vi "GEA_Brute_Force_SM.vi"(0 "ComPort":refnum<visa-resource-name>="COM1", 1 "Destination Address":u8=96 format="%.0x", 2 "Source Address":u8=128 format="%.0x", 5 "Command":u8(ring)=15 items=["CMD_WRITE_SETPOINTS", "RQST_NON_CRIT_VERSION", "RQST_CRIT_VERSION", "RQST_EEPROM_VERSION", "RQST_T2_RESISTANCE", "RQST_T3A_RESISTANCE", "RQST_T3B_RESISTANCE", "RQST_T4_RESISTANCE", "RQST_T5_RESISTANCE", "RQST_IDLB_RESISTANCE", "RQST_MODE_SELECT_RESISTANCE", "RQST_STATUS INFO", "RQST_SS_FAULT_COUNTS", "RQST_OTHER_FAULT_COUNTS", "CMD_CLEAR_FAULT_COUNTS", "RQST_HYPERTERM_OUTPUT_DATA", "RQST_READ_PERSONALITY", "RQST_DSM_OVERRIDE_STATUS", "RQST_STATUS_QUERY", "RQST_HEM_KWH_DATA", "RQST_SERVICE_ERROR_CODES", "RQST_OVERRIDE_STATUS", "CMD_CLEAR_OVERRIDE_STATUS", "CMD_CLEAR_ENERGY_USAGE_CTRS", "CMD_COMP_OFF", "CMD_UE_2_SECONDS", "CMD_LE_2_SECONDS", "CMD_COMP_ON", "CMD_HP_RUN_6MIN", "RQST_TEMP_RANGE", "RQST_VACATION_RANGE", "RQST_STD_ELEC_RANGE", "RQST_WATER_CAPACITY", "CMD_CANCEL_EEV_POSITION", "RQST_SUPPORTED_MODES", "CMD_CONTROL_FAN1", "CMD_EEV_POSITION", "CMD_SET_EEV_START_POSITION", "CMD_SET_EEV_STOP_POSITION", "CMD_UPDATE_DSM_LEVEL", "CMD_SET_PID_I_DENOMINATOR", "CMD_SET_PID_I_NUMERATOR", "RQST_DATA_FROM_MEMORY", "CMD_OVERRIDE_STATUS_CHANGED", "CMD_SET_PID_P_DENOMINATOR", "CMD_SET_PID_P_NUMERATOR", "CMD_SET_PID_RUN_SH_TARGET", "CMD_SET_PID_START_DWELL_TIME", "CMD_SET_PID_TRANSITION_TIME", "CMD_SET_PID_TRANS_SH_TARGET", "CMD_SET_PID_UPDATE_RATE", "RQST_DATA_FROM_DATA_FLASH", "CMD_DSM_OVERRIDES", "CMD_UPDATE_MODE", "CMD_UPDATE_SPECIAL_OPERATION", "CMD_SET_CURRENTS", "CMD_RESET_FILTER_TIMES", "CMD_TURN_ON_DLB", "RQST_PID_PARAMETERS", "CMD_CHECK_CRC", "CMD_ENTER_FACT_MODE", "CMD_RESET", "CMD_RESTORE_EEPROM_DEFAULTS"], 7 "Command Data":u8[](array[numeric]) format="%02x", 9 "InitSerial?":bool=TRUE, 11 "Error In":errorcluster) -> (4 "WriteACK":bool, 6 "Read_ACK":bool, 8 "DataReturned":u8[](array[numeric]) format="%.0x", 14 "CRC Match":bool, 15 "Error Out":errorcluster)   [LabVIEW 2009]
uses:
  <vilib>/Instr/_visa.llb/VISA Configure Serial Port (Instr).vi
  HEWH Error Enumeration.ctl
panel:
  out "tStart":i32
  out "Diff Time":i32[](array[numeric])
  out "Serial Settings:Number of Bytes at Serial Port":u32
  out "Time Array":i32[](array[numeric])
  out "ACK(E1?)":u8[](array[numeric]) format="%.0x"
  out "Local?":bool
  out "State Array":string[](array[string])
  out "CRCRead":u8[](array[numeric]) format="%.0x"
  out "Command":u8[](array[numeric])=[226, 96, 8, 128, 86, 123, 137, 227] format="%.0x"
  in  "Send HEWH Cmd":bool
  in  "Write Rand":bool
  in  "Random Data":u8[](array[numeric]) format="%.0x"
  out "WriteOK":bool
  out "ReadArray":u8[](array[numeric]) format="%.0x"
  in  "OK":bool
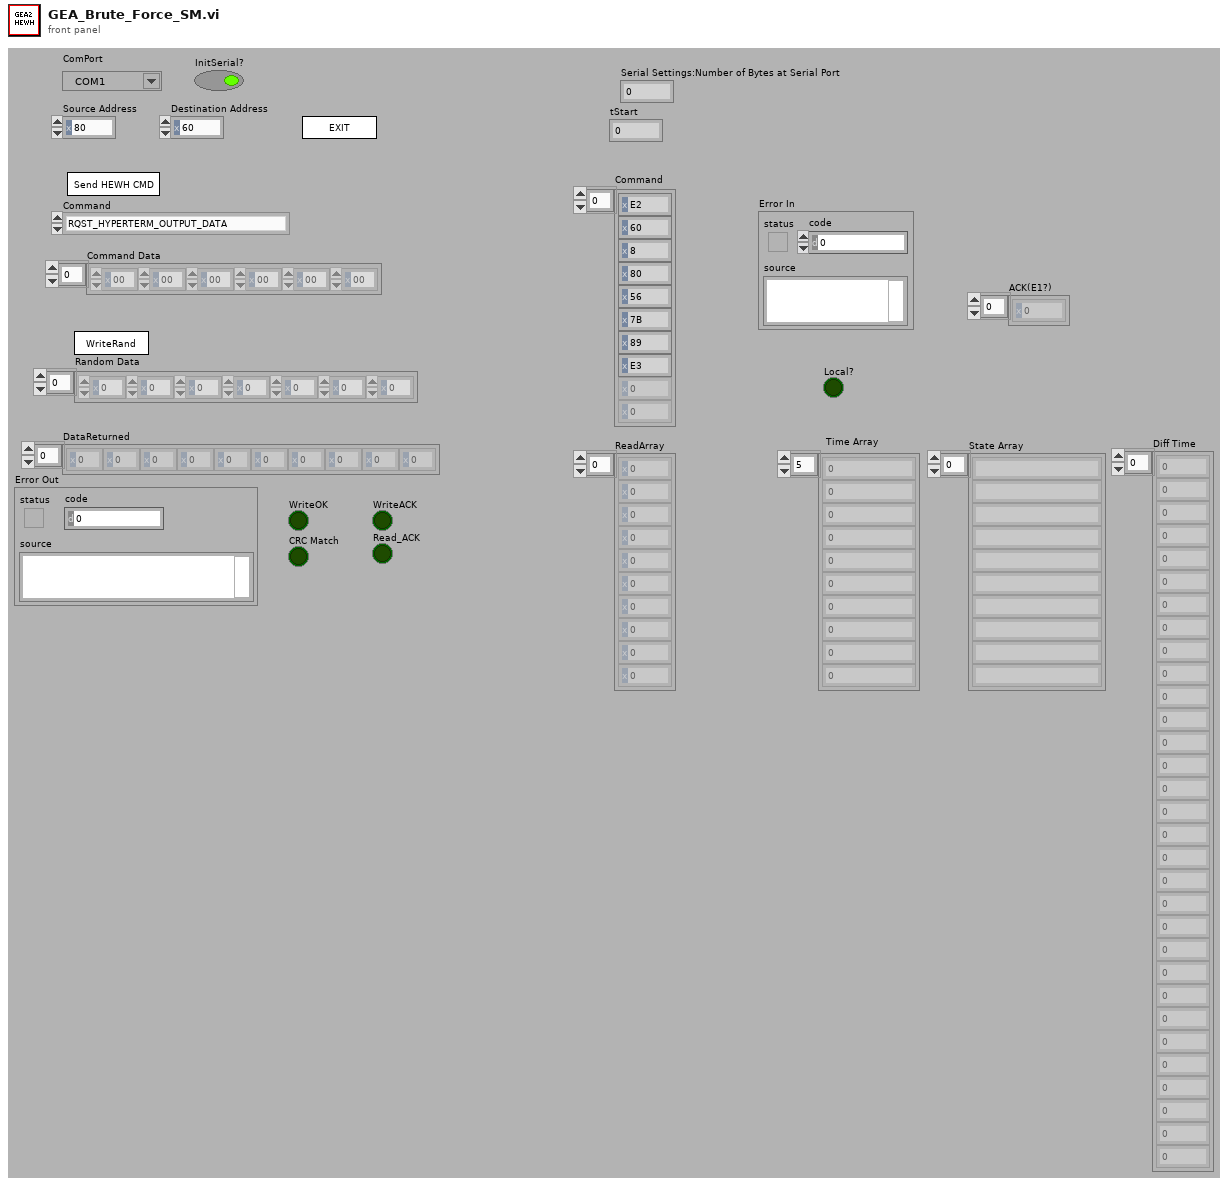
[diagram p1: front panel]
types:
  T1 = enum32{"invalid app kind", "Development System", "Run Time System", "Student Edition", "Embedded LabVIEW", "Evaluation", "Custom"}
  T2 = enum32{"Invalid", "Standard", "Closed", "Hidden", "Minimized", "Maximized"}
  T3 = typedef "HEWH Error Enumeration.ctl" = enum16{"No Error", "GEA2 Send ACK Mismatch", "GEA2 STX", "GEA2 ETX", "GEA2 CRC Mismatch", "GEA2 ReadACK", "RTD In Range Error", "Fail Mean Tank Temp"}
  T4 = cluster{"Core":cluster{"Current VI Reference":refnum<vi>, "Close Panel on Exit?":bool}, "ComPort":refnum<visa-resource-name>, "ReadArray":u8[], "CRCArray":u8[], "Bytes Remaining":u8, "CRCRead":u8[], "Error Out Flag":bool, "CRC":bool}
  T5 = cluster{"Current VI Reference":refnum<vi>, "Close Panel on Exit?":bool}
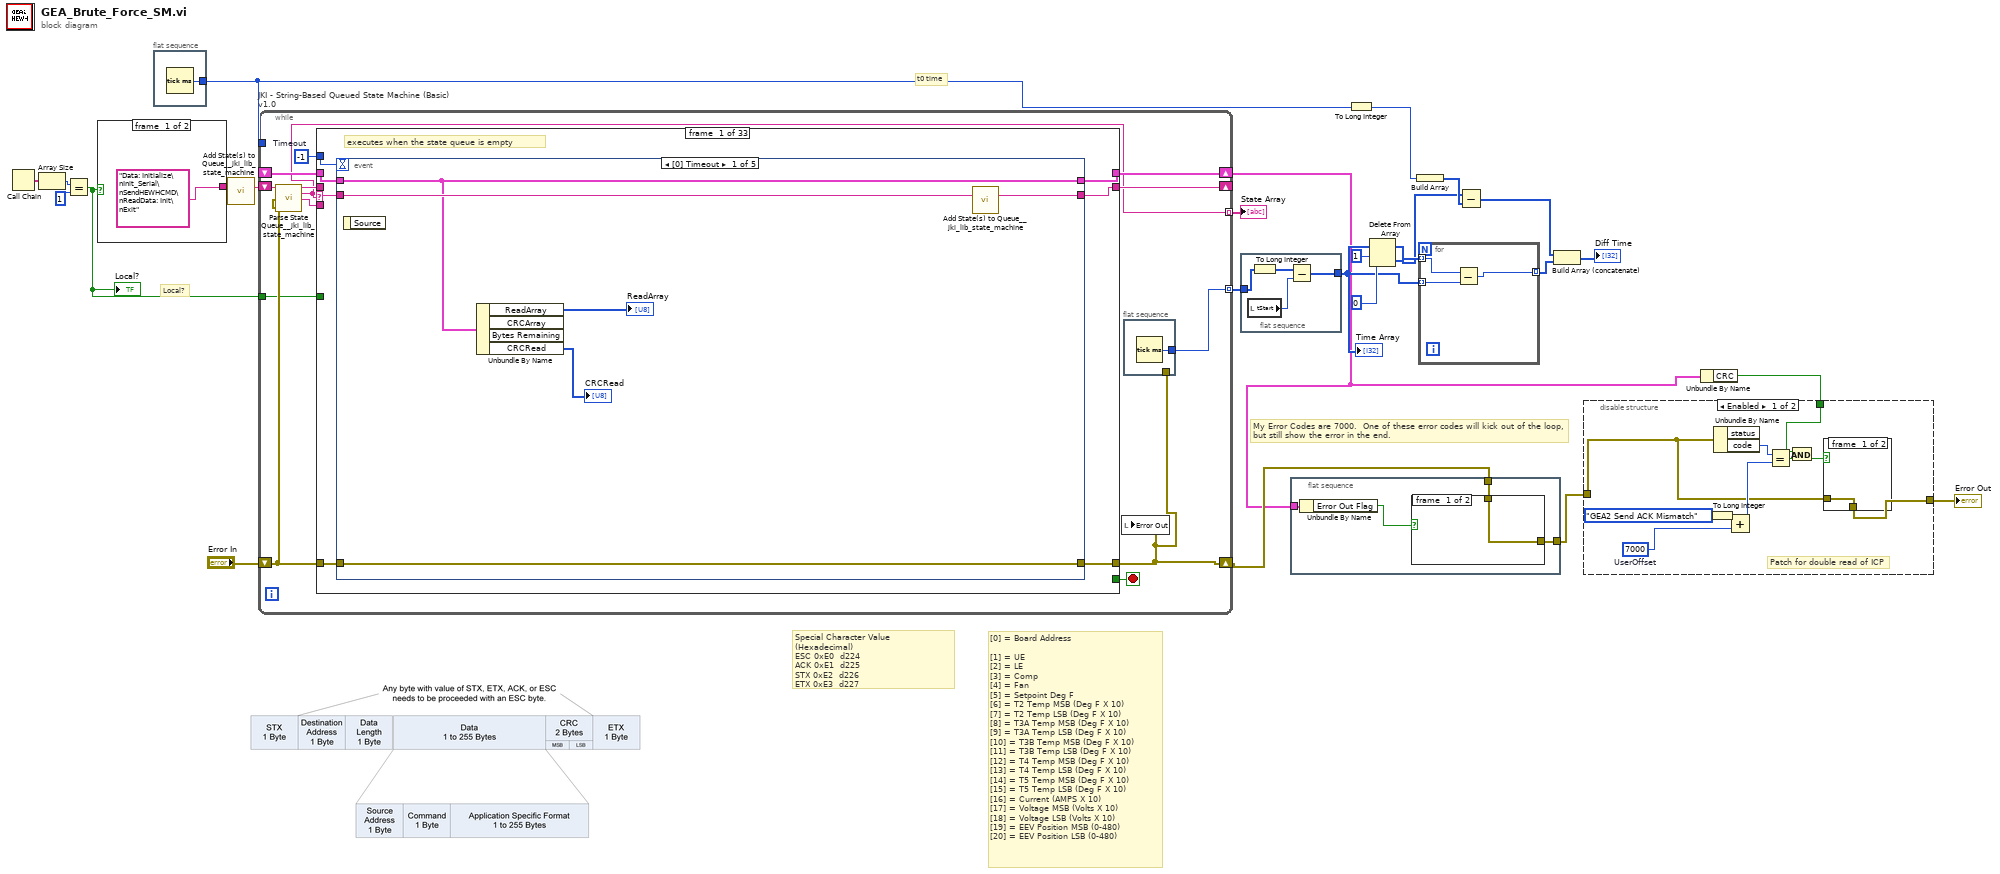
[diagram p0: block diagram]
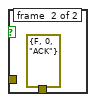
[diagram p2: hidden frame]
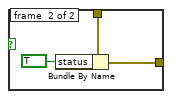
[diagram p4: hidden frame]
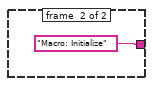
[diagram p5: hidden frame]
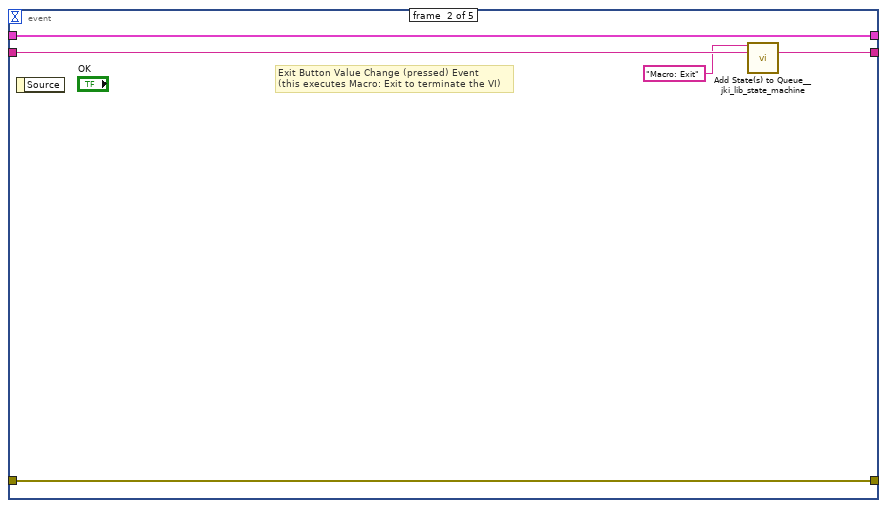
[diagram p6: hidden frame]
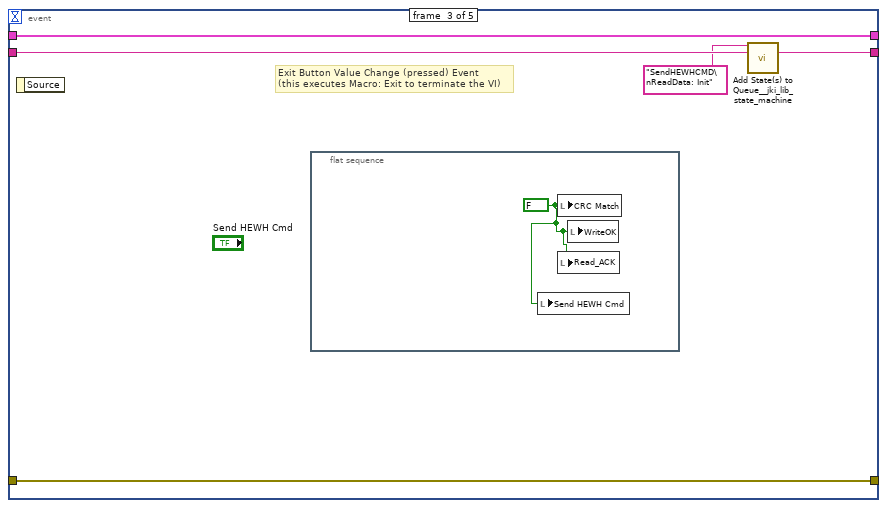
[diagram p7: hidden frame]
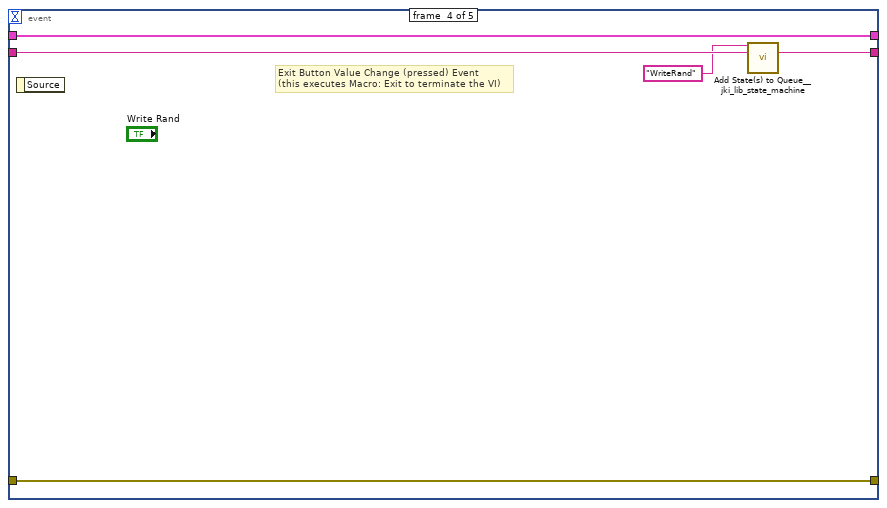
[diagram p8: hidden frame]
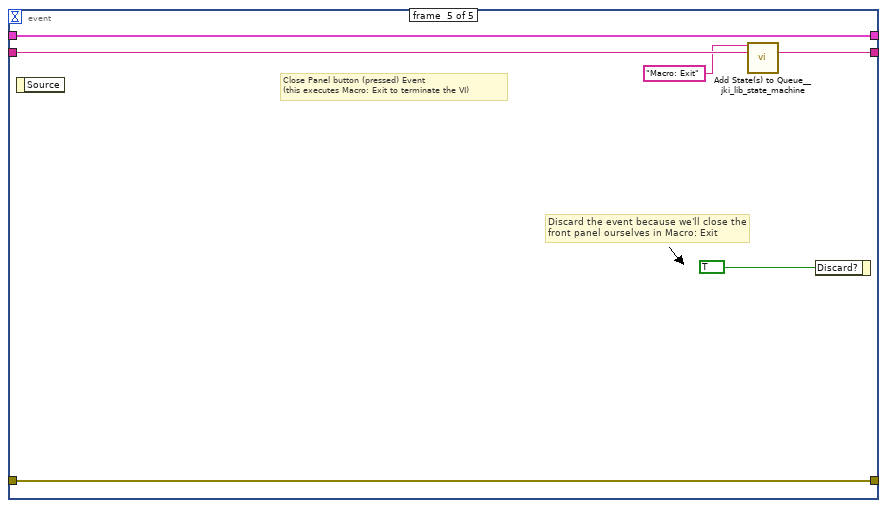
[diagram p9: hidden frame]
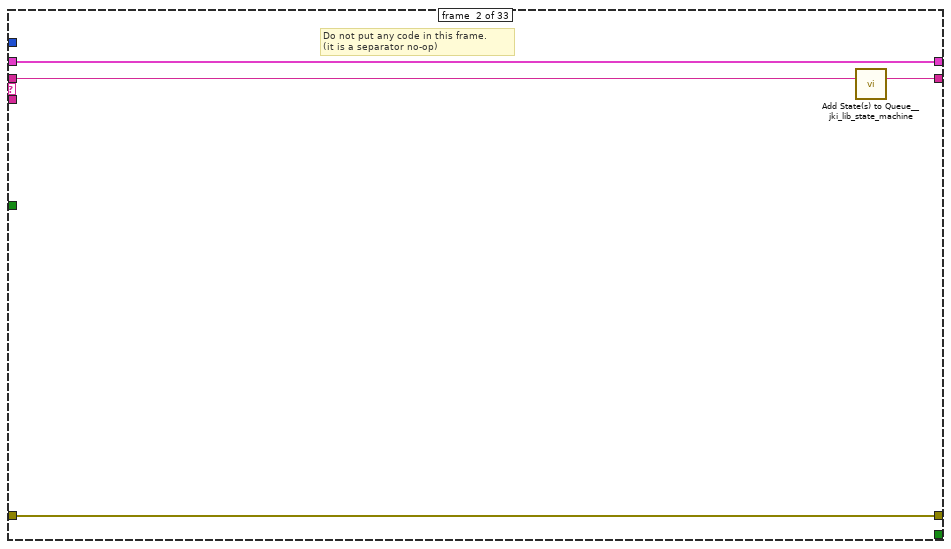
[diagram p10: hidden frame]
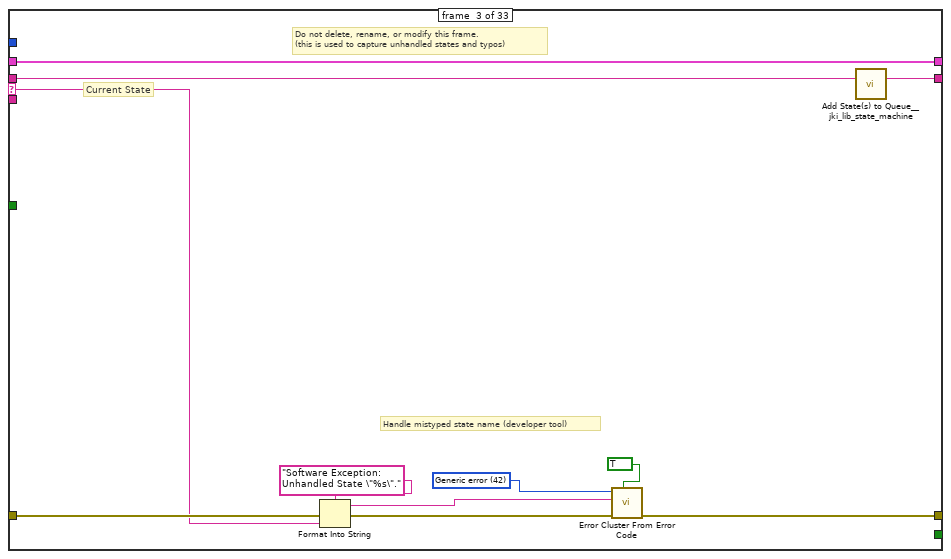
[diagram p11: hidden frame]
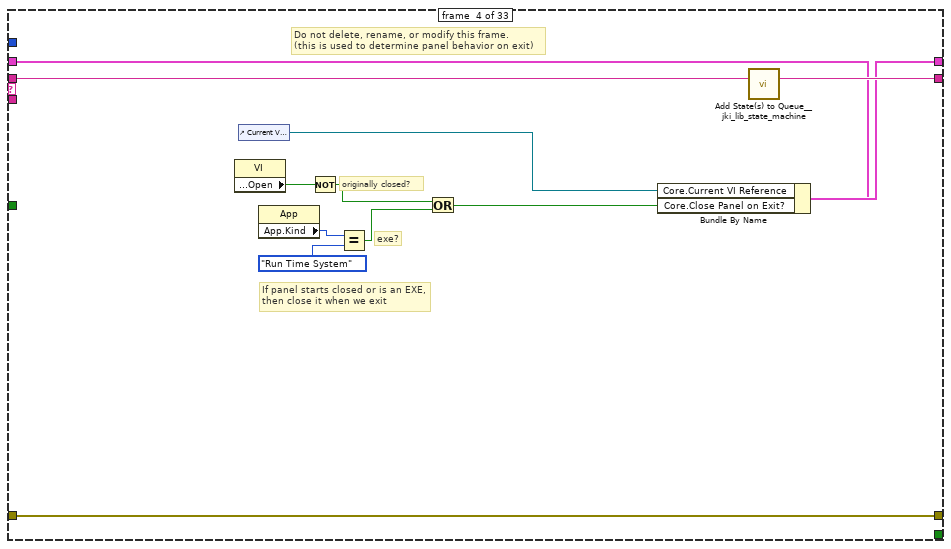
[diagram p12: hidden frame]
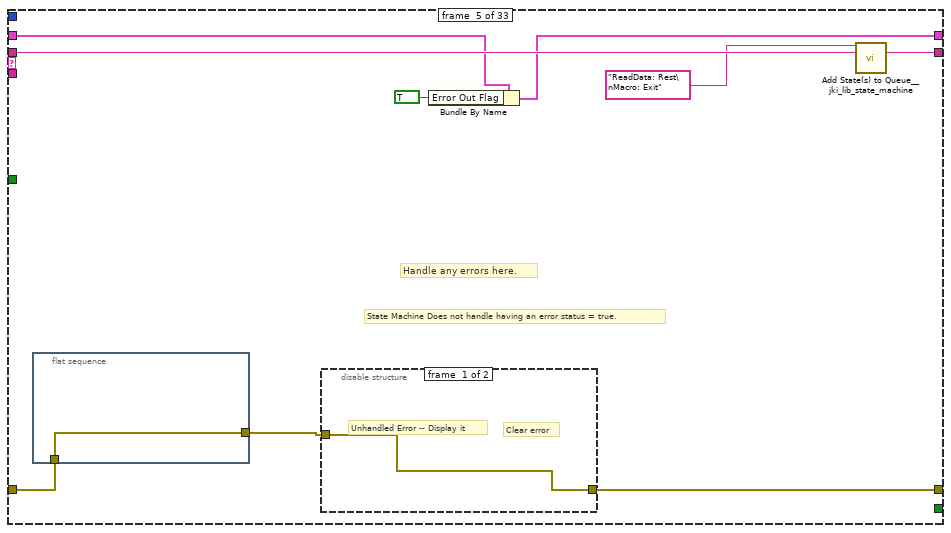
[diagram p13: hidden frame]
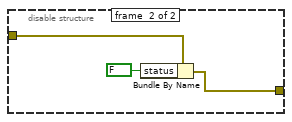
[diagram p14: hidden frame]
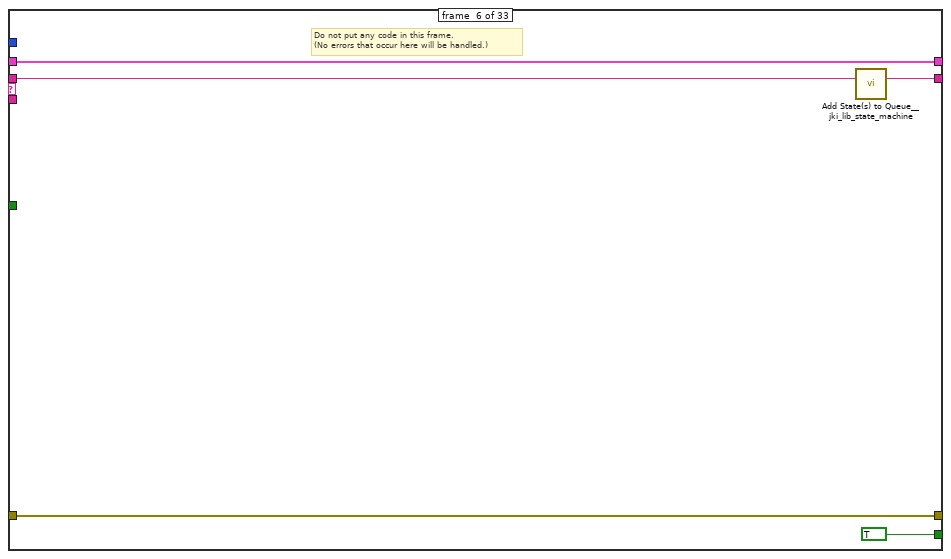
[diagram p15: hidden frame]
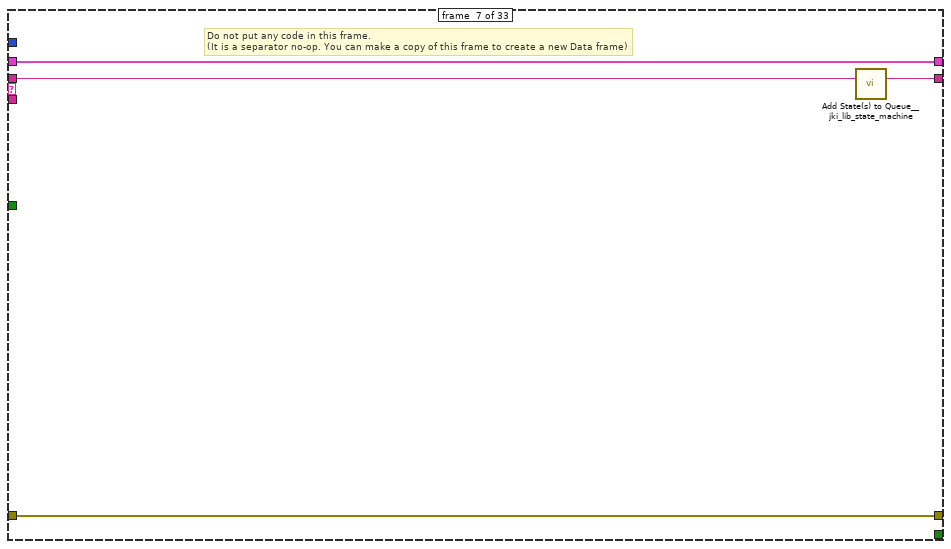
[diagram p16: hidden frame]
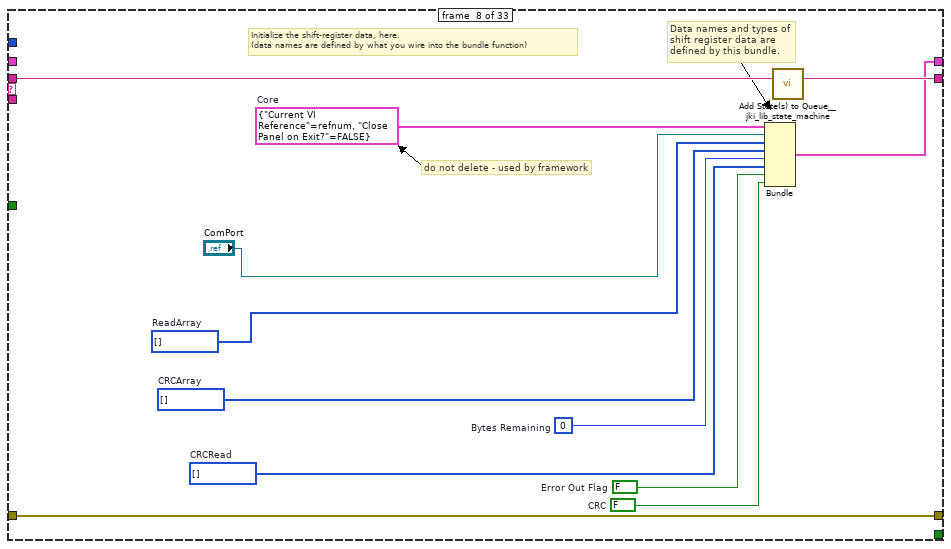
[diagram p17: hidden frame]
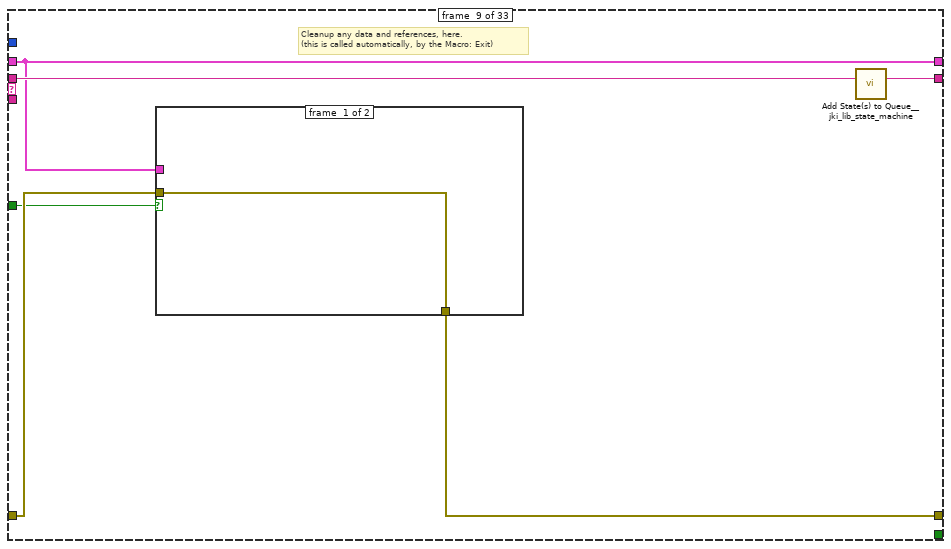
[diagram p18: hidden frame]
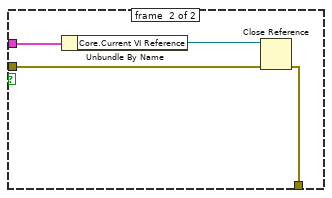
[diagram p19: hidden frame]
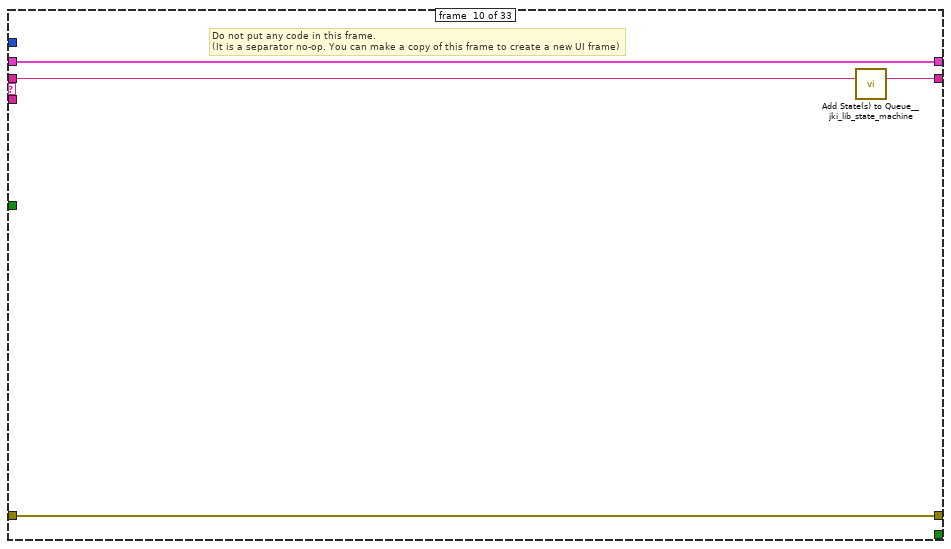
[diagram p20: hidden frame]
diagram:
  # "t0 time"
  # "My Error Codes are 7000.  One of these error codes will kick out of the loop,\nbut still show the error in the end."
  # "Local?"
  # "Special Character\tValue (Hexadecimal)\nESC\t0xE0  d224\nACK\t0xE1  d225\nSTX\t0xE2  d226\nETX\t0xE3  d227"
  # "[0] = Board Address\n\n[1] = UE\n[2] = LE\n[3] = Comp\n[4] = Fan\n[5] = Setpoint Deg F\n[6] = T2 Temp MSB (Deg F X 10)\n[7] = T2 Temp LSB (Deg F X 10)\n[8] = T3A Temp MSB (Deg F X 10)\n[9] = T3A Temp LSB (Deg F X 10)\n[10] = T3B Temp MSB (Deg F X 10)\n[11] = T3B Temp LSB (Deg F X 10)\n[12] = T4 Temp MSB (Deg F X 10)\n[13] = T4 Temp LSB (Deg F X 10)\n[14] = T5 Temp MSB (Deg F X 10)\n[15] = T5 Temp LSB (Deg F X 10)\n[16] = Current (AMPS X 10)\n[17] = Voltage MSB (Volts X 10)\n[18] = Voltage LSB (Volts X 10)\n[19] = EEV Position MSB (0-480)\n[20] = EEV Position LSB (0-480)"
  n1 = Call Chain() -> (call chain=w22:string[])
  n2 = Array Size(array=w22) -> (size(s)=w21:i32)
  n3 = Equal?(x=w21, y=1) -> (x = y?=w19:bool)
  "Local?" <- w19
  n4 = case shown="False" w19 {
    tunnel: ["Data: Initialize\nInit_Serial\nSendHEWHCMD\nReadData: Init\nExit" "Macro: Initialize"] -> w24
    frame #0 {
    }
    frame #1 {
    }
  }
  n5 = flat-sequence {
    tunnel: [w28] -> w9
    frame #0 {
      n6 = Tick Count (ms)() -> (millisecond timer value=w28:u32)
    }
  }
  n7 = call <vilib>:"Add State(s) to Queue__jki_lib_state_machine.vi"("State(s) in (\"\")"=w24) -> ("States Out"=w25:string)  [unwired: 14 in]
  n8 = while "JKI - String-Based Queued State Machine (Basic) v1.0" {
    shift-right: [w37] -> w2
    shift-left: _ -> [w36]
    shift-right: [w30] -> w18
    shift-left: "Error In" -> [w34]
    shift-right: [w32] -> _
    shift-left: w25 -> [w39]
    tunnel: w19 -> [w33]
    tunnel: [w31] -> w17 mode=indexing
    tunnel: [w29] -> w12 mode=indexing
    tunnel: w9 -> [_]
    stop <- w38 stop-if-true
    w35 = -1  # Timeout
    n9 = call <vilib>:"Parse State Queue__jki_lib_state_machine.vi"("State Queue"=w39, "Error In (no error)"=w34) -> ("Remaining States"=w41:string, "Current State"=w31:string, "Arguments"=w40:string)  [unwired: 11 in]
    n10 = case shown="\"ReadData: CheckCRC\"" w31 {
      selector: w31 -> [_ _ w82 _ _ _ _ _ _ _ _ _ _ _ _ _ _ _ _ _ _ _ _ _ _ _ _ _ _ _ _ _ _]
      tunnel: w41 -> [w49 w81 w86 w104 w113 w123 w127 w139 w145 w154 w159 w165 w176 w202 w207 w217 w221 w229 w304 w342 w357 w364 w382 w413 w460 w504 w542 w576 w600 w625 w650 w669 w694]
      tunnel: w40 -> [_ _ _ _ _ _ _ _ _ _ _ w160 w170 _ _ _ _ _ _ _ _ _ _ _ _ _ _ _ _ _ _ _ _]
      tunnel: w36 -> [w47 w78 w84 w95 w107 w121 w124 _ w142 w151 w157 w163 w172 w199 w204 w214 w218 w226 w302 w340 w354 w361 w378 w411 w457 w501 w539 w574 w591 w620 w645 w665 w692]
      tunnel: [w46 w79 w88 w101 w111 w120 w125 w136 w140 w152 w156 w161 w173 w200 w205 w215 w219 w227 w299 w336 w355 w362 w368 w403 w450 w496 w523 w560 w595 w615 w640 w667 w678] -> w30
      tunnel: w34 -> [w45 w79 w87 w101 w109 w120 w125 w136 w143 w152 w156 w162 w174 w200 w205 w215 w219 w224 w300 w337 w355 w362 w371 w405 w452 w497 w535 w570 w597 w618 w643 w667 w691]
      tunnel: [w48 w80 w85 w103 w112 w122 w126 w138 w144 w153 w158 w164 w175 w201 w206 w216 w220 w228 w303 w341 w356 w363 w381 w412 w459 w503 w541 w575 w599 w624 w649 w668 w693] -> w32
      tunnel: [_ _ _ _ _ TRUE _ _ _ _ _ _ _ _ _ _ _ _ _ _ _ _ _ _ _ _ _ _ _ _ _ _ _] -> w38
      tunnel: [w44 w78 w84 w102 w106 w121 w124 w137 w142 w151 w157 w163 w172 w199 w204 w214 w218 w225 w302 w340 w354 w360 w377 w410 w456 w500 w538 w573 w590 w619 w644 w664 w692] -> w37
      tunnel: w35 -> [w43 _ _ _ _ _ _ _ _ _ _ _ _ _ _ _ _ _ _ _ _ _ _ _ _ _ _ _ _ _ _ _ _]
      tunnel: w33 -> [_ _ _ _ _ _ _ _ w141 _ _ _ _ _ _ _ _ w223 _ _ _ _ _ _ _ _ _ _ _ _ _ _ _]
      frame #0 {
        # "executes when the state queue is empty"
        n11 = event shown="[0] Timeout" {
          selector: _ -> [_ _ _ _ _]
          dyn-events: _ -> [_ _ _ _ _]
          timeout: w43 -> [_ _ _ _ _]
          tunnel: w49 -> [w55 w60 w65 w71 w77]
          tunnel: [w54 w59 w64 w70 w76] -> w48
          tunnel: w47 -> [w52 w57 w62 w68 w74]
          tunnel: [w53 w58 w63 w69 w75] -> w46
          tunnel: w45 -> [w53 w58 w63 w69 w75]
          tunnel: [w52 w57 w62 w68 w74] -> w44
          event #0 {
            n12 = event-data() -> ()  [unwired: 1 in, 1 out]
            n13 = Unbundle By Name(w52) -> ("ReadArray"=→"ReadArray":u8[], "CRCRead"=→"CRCRead":u8[])  [unwired: 2 out]
            n14 = call <vilib>:"Add State(s) to Queue__jki_lib_state_machine.vi"("State(s) in (\"\")"=w55) -> ("States Out"=w54:string)  [unwired: 14 in]
          }
          event #1 {
            # "Exit Button Value Change (pressed) Event\n(this executes Macro: Exit to terminate the VI)"
            n15 = event-data() -> ()  [unwired: 1 in, 1 out]
            n16 = call <vilib>:"Add State(s) to Queue__jki_lib_state_machine.vi"("State(s) in Front (\"\")"="Macro: Exit", "State(s) in (\"\")"=w60) -> ("States Out"=w59:string)  [unwired: 13 in]
          }
          event #2 {
            # "Exit Button Value Change (pressed) Event\n(this executes Macro: Exit to terminate the VI)"
            n17 = event-data() -> ()  [unwired: 1 in, 1 out]
            n18 = flat-sequence {
              frame #0 {
                w66 = FALSE ("CRC Match")
                n19 = local write "Send HEWH Cmd"(w66) -> ()
                n20 = local write "CRC Match"(w66) -> ()
                n21 = local write "Read_ACK"(w66) -> ()
                n22 = local write "WriteOK"(w66) -> ()
              }
            }
            n23 = call <vilib>:"Add State(s) to Queue__jki_lib_state_machine.vi"("State(s) in Front (\"\")"="SendHEWHCMD\nReadData: Init", "State(s) in (\"\")"=w65) -> ("States Out"=w64:string)  [unwired: 13 in]
          }
          event #3 {
            # "Exit Button Value Change (pressed) Event\n(this executes Macro: Exit to terminate the VI)"
            n24 = event-data() -> ()  [unwired: 1 in, 1 out]
            n25 = call <vilib>:"Add State(s) to Queue__jki_lib_state_machine.vi"("State(s) in Front (\"\")"="WriteRand", "State(s) in (\"\")"=w71) -> ("States Out"=w70:string)  [unwired: 13 in]
          }
          event #4 {
            # "Discard the event because we'll close the front panel ourselves in Macro: Exit"
            # "Close Panel button (pressed) Event\n(this executes Macro: Exit to terminate the VI)"
            n26 = event-data() -> ()  [unwired: 1 in, 1 out]
            n27 = call <vilib>:"Add State(s) to Queue__jki_lib_state_machine.vi"("State(s) in Front (\"\")"="Macro: Exit", "State(s) in (\"\")"=w77) -> ("States Out"=w76:string)  [unwired: 13 in]
            n28 = event-data("Discard?"=TRUE) -> ()  [unwired: 1 in, 1 out]
          }
        }
      }
      frame #1 {
        # "Do not put any code in this frame.\n(it is a separator no-op)"
        n29 = call <vilib>:"Add State(s) to Queue__jki_lib_state_machine.vi"("State(s) in (\"\")"=w81) -> ("States Out"=w80:string)  [unwired: 14 in]
      }
      frame #2 {
        w91 = 42 items=["No error", "Argument error", "Memory is full", "Out of zone", "End of file", "File already open", "Generic file I/O error", "File not found", "File permission error", "Disk is full", "Duplicate path", "Too many files open", "System feature not enabled", "Resource file not found", "Cannot add resource", "Resource not found", "Image not found", "Image memory error", "Pen does not exist", "Config type invalid", "Config token not found", "Config parse error", "Config memory error", "Bad external code format", "Bad external code offset", "External code not present", "Null window", "Destroy window error", "Null menu", "Print aborted", "Bad print record", "Print driver error", "Windows error during printing", "Memory error during printing", "Print dialog error", "Generic print error", "Invalid device refnum", "Device not found", "Device parameter error", "Device unit error", "Cannot open device", "Device call aborted", "Generic error", "Cancelled by user", "Object ID too low", "Object ID too high", "Object not in heap", "Unknown heap", "Unknown object (invalid DefProc)", "Unknown object (DefProc not in table)", "Message out of range", "Invalid (null) method", "Unknown message", "Manager call not supported", "Bad address", "Network operation in progress", "Network operation timed out", "Connection is busy", "Network attribute not supported", "Network error", "Address in use", "System out of memory", "Connection aborted", "Connection refused", "Not connected", "Already connected", "Connection closed", "Initialization error (interapplication manager)", "Bad occurrence", "Wait on unbound occurrence handler", "Occurrence queue overflow", "Datalog type conflict", "Unused", "Unrecognized type (interapplication manager)", "Memory corrupt", "Failed to make temporary DLL", "Old CIN version", "Drag socket not found", "Failed to load drop-object", "Failed to register OLE object", "Failed to release OLE object", "Format specifier type mismatch", "Unknown format specifier", "Too few format specifiers", "Too many format specifiers", "Scan failed", "Newer CIN version", "Error converting to variant", "Runtime menu error", "Password tampered", "Variant attribute not found", "Incompatible variant data type", "Event data is not available", "Event Store is not present", "Occurrence is not found", "Event Queue is not created", "Event info is not available", "Refnum passed is NULL", "Error retrieving Class GUID", "Error retrieving CoClass GUID", "Error retrieving TypeLib GUID.", "Bad built application magic bytes.", "Specific driver is different from the specific driver associated with the Logical Name.", "There is no session opened to the class driver.", "Max Error", "MAX - Error with config objects", "MAX - Error loading configuration", "MAX - Group not supported"]
        # "Current State"
        # "Do not delete, rename, or modify this frame.\n(this is used to capture unhandled states and typos)"
        # "Handle mistyped state name (developer tool)"
        n30 = Format Into String(format string="Software Exception: Unhandled State \"%s\"." ("message"), error in=w87, w82) -> (resulting string=w90:string, error out=w89:errorcluster)  [unwired: 1 in]
        n31 = call <vilib>:"Error Cluster From Error Code.vi"("show call chain? (False)"=TRUE, "error in (no error)"=w89, "error message (\"\")"=w90, "error code (0)"=w91) -> ("error out"=w88:errorcluster)  [unwired: 5 in]
        n32 = call <vilib>:"Add State(s) to Queue__jki_lib_state_machine.vi"("State(s) in (\"\")"=w86) -> ("States Out"=w85:string)  [unwired: 14 in]
      }
      frame #3 {
        # "Do not delete, rename, or modify this frame.\n(this is used to determine panel behavior on exit)"
        # "originally closed?"
        # "exe?"
        # "If panel starts closed or is an EXE, then close it when we exit"
        n33 = property class="VI"() -> ("Front Panel.Open"=w100:bool)  [unwired: 2 in, 2 out]
        n34 = control-ref of="Current VI Reference"() -> (w93:refnum<vi>)
        n35 = property class="App"() -> ("App.Kind"=w99:T1)  [unwired: 2 in, 2 out]
        n36 = Not(x=w100) -> (.not. x?=w97:bool)
        n37 = Equal?(x=w99, y=T1."Run Time System" ("Application:Kind")) -> (x = y?=w96:bool)
        n38 = Or(x=w97, y=w96) -> (x .or. y?=w94:bool)
        n39 = Bundle By Name(cluster=w95, "Core.Current VI Reference"=w93, "Core.Close Panel on Exit?"=w94) -> (w102:T4)
        n40 = call <vilib>:"Add State(s) to Queue__jki_lib_state_machine.vi"("State(s) in (\"\")"=w104) -> ("States Out"=w103:string)  [unwired: 14 in]
      }
      frame #4 {
        # "State Machine Does not handle having an error status = true."
        # "Handle any errors here."
        n41 = flat-sequence {
          tunnel: w109 -> [w114]
          tunnel: [w114] -> w108
          frame #0 {
          }
        }
        n42 = disable-structure shown="Enabled" {
          disable-tunnel: [w115 w117] -> w111
          disable-tunnel: w108 -> [w115 w118]
          frame #0 {
            # "Unhandled Error -- Display it"
            # "Clear error"
          }
          frame #1 {
            n43 = Bundle By Name(cluster=w118, "status"=FALSE) -> (w117:errorcluster)
          }
        }
        n44 = Bundle By Name(cluster=w107, "Error Out Flag"=TRUE) -> (w106:T4)
        n45 = call <vilib>:"Add State(s) to Queue__jki_lib_state_machine.vi"("State(s) in Front (\"\")"="ReadData: Rest\nMacro: Exit", "State(s) in (\"\")"=w113) -> ("States Out"=w112:string)  [unwired: 13 in]
      }
      frame #5 {
        # "Do not put any code in this frame.\n(No errors that occur here will be handled.)"
        n46 = call <vilib>:"Add State(s) to Queue__jki_lib_state_machine.vi"("State(s) in (\"\")"=w123) -> ("States Out"=w122:string)  [unwired: 14 in]
      }
      frame #6 {
        # "Do not put any code in this frame.\n(It is a separator no-op. You can make a copy of this frame to create a new Data frame)"
        n47 = call <vilib>:"Add State(s) to Queue__jki_lib_state_machine.vi"("State(s) in (\"\")"=w127) -> ("States Out"=w126:string)  [unwired: 14 in]
      }
      frame #7 {
        w128 = FALSE  # CRC
        w129 = FALSE  # Error Out Flag
        w130 = u8[] []  # CRCRead
        w131 = u8 0  # Bytes Remaining
        w132 = u8[] []  # CRCArray
        w133 = u8[] []  # ReadArray
        w135 = T5 {"Current VI Reference"=refnum, "Close Panel on Exit?"=FALSE}  # Core
        # "do not delete - used by framework"
        # "Data names and types of shift register data are defined by this bundle."
        # "Initialize the shift-register data, here.\n(data names are defined by what you wire into the bundle function)"
        n48 = Bundle("Core"=w135, "ComPort"="ComPort", "ReadArray"=w133, "CRCArray"=w132, "Bytes Remaining"=w131, "CRCRead"=w130, "Error Out Flag"=w129, "CRC"=w128) -> (w137:T4)  [unwired: 1 in]
        n49 = call <vilib>:"Add State(s) to Queue__jki_lib_state_machine.vi"("State(s) in (\"\")"=w139) -> ("States Out"=w138:string)  [unwired: 14 in]
      }
      frame #8 {
        # "Cleanup any data and references, here.\n(this is called automatically, by the Macro: Exit)"
        n50 = case shown="True" w141 {
          tunnel: w143 -> [w146 w149]
          tunnel: [w146 w148] -> w140
          tunnel: w142 -> [_ w147]
          frame #0 {
          }
          frame #1 {
            n51 = Unbundle By Name(w147) -> ("Core.Current VI Reference"=w150:refnum<vi>)
            n52 = Close Reference(reference=w150, error in (no error)=w149) -> (error out=w148:errorcluster)
          }
        }
        n53 = call <vilib>:"Add State(s) to Queue__jki_lib_state_machine.vi"("State(s) in (\"\")"=w145) -> ("States Out"=w144:string)  [unwired: 14 in]
      }
      frame #9 {
        # "Do not put any code in this frame.\n(It is a separator no-op. You can make a copy of this frame to create a new UI frame)"
        n54 = call <vilib>:"Add State(s) to Queue__jki_lib_state_machine.vi"("State(s) in (\"\")"=w154) -> ("States Out"=w153:string)  [unwired: 14 in]
      }
      frame #10 {
        w155 = FALSE ("CRC Match")
        # "Initialize the User Interface, here.\n(this is called automatically, by the Macro: Init)"
        n55 = local write "CRC Match"(w155) -> ()
        n56 = local write "WriteOK"(w155) -> ()
        n57 = local write "WriteACK"(w155) -> ()
        n58 = local write "Send HEWH Cmd"(w155) -> ()
        n59 = call <vilib>:"Add State(s) to Queue__jki_lib_state_machine.vi"("State(s) in (\"\")"=w159) -> ("States Out"=w158:string)  [unwired: 14 in]
      }
      frame #11 {
        # "Argument"
        # "Set and Unset Cursor Busy.\n(Usage: \"UI: Cursor Set >> Busy|Idle\")"
        n60 = case shown="\"Idle\", Default" w160 {
          tunnel: w162 -> [w167 w169]
          tunnel: [w166 w168] -> w161
          frame #0 {
            n61 = call <vilib>:"Unset Busy.vi"("error in (no error)"=w167) -> ("error out"=w166:errorcluster)  [unwired: 10 in]
          }
          frame #1 {
            n62 = call <vilib>:"Set Busy.vi"("error in (no error)"=w169) -> ("error out"=w168:errorcluster)  [unwired: 9 in, 1 out]
          }
        }
        n63 = call <vilib>:"Add State(s) to Queue__jki_lib_state_machine.vi"("State(s) in (\"\")"=w165) -> ("States Out"=w164:string)  [unwired: 14 in]
      }
      frame #12 {
        # "Argument"
        # "Set Front Panel Open or Closed\n(Usage: \"UI: Front Panel State >> Open|Close\")"
        n64 = Unbundle By Name(w172) -> ("Core.Current VI Reference"=w171:refnum<vi>)
        n65 = case shown="\"Close\"" w170 {
          tunnel: w174 -> [w180 w193]
          tunnel: [w182 w194] -> w173
          tunnel: w171 -> [w181 w191]
          frame #0 {
            n66 = property class="VI"(reference=w181, error in=w180) -> (reference out=w178:refnum<vi>, error out=w179:errorcluster, "Front Panel.Open"=w177:bool)
            n67 = case shown="False" w177 {
              tunnel: [w185 w188] -> w182
              tunnel: w179 -> [w184 w188]
              tunnel: w178 -> [w183 _]
              frame #0 {
                n68 = invoke class="VI" method="FP.Open"(reference=w183, error in=w184, "Activate"=TRUE, "State"=T2."Standard") -> (error out=w185:errorcluster)  [unwired: 1 in, 4 out]
              }
              frame #1 {
              }
            }
          }
          frame #1 {
            n69 = property class="VI"(reference=w191, error in=w193) -> (reference out=w190:refnum<vi>, error out=w192:errorcluster, "Front Panel.Open"=w189:bool)
            n70 = case shown="True" w189 {
              tunnel: [w195 w198] -> w194
              tunnel: w192 -> [w195 w197]
              tunnel: w190 -> [_ w196]
              frame #0 {
              }
              frame #1 {
                n71 = invoke class="VI" method="FP.Close"(reference=w196, error in=w197) -> (error out=w198:errorcluster)  [unwired: 1 in, 2 out]
              }
            }
          }
        }
        n72 = call <vilib>:"Add State(s) to Queue__jki_lib_state_machine.vi"("State(s) in (\"\")"=w176) -> ("States Out"=w175:string)  [unwired: 14 in]
      }
      frame #13 {
        # "Do not put any code in this frame.\n(It is a separator no-op. You can make a copy of this frame to create a new Macro frame)"
        n73 = call <vilib>:"Add State(s) to Queue__jki_lib_state_machine.vi"("State(s) in (\"\")"=w202) -> ("States Out"=w201:string)  [unwired: 14 in]
      }
      frame #14 {
        w203 = "Data: Initialize\nInitialize Core Data\nUI: Initialize\nUI: Front Panel State >> Open\nInit_Serial"  # Data: Initialize Initialize Core Data UI: Initialize UI: Front Panel State >> Open Init_Serial
        # "Initialization Macro\n(This is called once, when the VI starts)"
        n74 = call <vilib>:"Add State(s) to Queue__jki_lib_state_machine.vi"("State(s) in Front (\"\")"=w203, "State(s) in (\"\")"=w207) -> ("States Out"=w206:string)  [unwired: 13 in]
      }
      frame #15 {
        # "Exit Macro\n(This is called once, when the VI exits)"
        n75 = Unbundle By Name(w214) -> ("Core.Close Panel on Exit?"=w213:bool)
        n76 = Select(t="UI: Front Panel State >> Close", s=w213, f="") -> (s? t:f=w210:string)
        n77 = call <vilib>:"Add State(s) to Queue__jki_lib_state_machine.vi"("State(s) in (\"\")"=w210, "State(s) at Back (\"\")"="Data: Cleanup\nExit") -> ("States Out"=w208:string)  [unwired: 13 in]
        n78 = call <vilib>:"Add State(s) to Queue__jki_lib_state_machine.vi"("State(s) in Front (\"\")"=w208, "State(s) in (\"\")"=w217) -> ("States Out"=w216:string)  [unwired: 13 in]
      }
      frame #16 {
        # "Template Separator\n(You can make a copy of, or modify, this frame)"
        n79 = call <vilib>:"Add State(s) to Queue__jki_lib_state_machine.vi"("State(s) in (\"\")"=w221) -> ("States Out"=w220:string)  [unwired: 14 in]
      }
      frame #17 {
        # "Your code here.\n(You can make a copy of, or modify, this frame)"
        n80 = case shown="True" "InitSerial?" {
          tunnel: [w235 w246] -> w227
          tunnel: w226 -> [w234 w251]
          tunnel: [w234 w250] -> w225
          tunnel: w224 -> [w236 w242]
          tunnel: w223 -> [_ _]
          frame #0 {
            n81 = Unbundle By Name(w234) -> ("ComPort"=w233:refnum<visa-resource-name>)
            n82 = property class="Instr"(reference=w233) -> (reference out=w230:refnum<visa-resource-name>, "Serial Settings:Number of Bytes at Serial Port"=w232:u32)  [unwired: 1 in, 1 out]
            n83 = Greater Than 0?(x=w232) -> (x > 0?=w231:bool)
            n84 = case shown="True" w231 {
              tunnel: w236 -> [w237 w240]
              tunnel: [w237 w239] -> w235
              tunnel: w230 -> [_ w238]
              frame #0 {
              }
              frame #1 {
                n85 = VISA Clear(VISA resource name=w238, error in (no error)=w240) -> (error out=w239:errorcluster)  [unwired: 1 out]
              }
            }
          }
          frame #1 {
            n86 = Unbundle By Name(w251) -> ("ComPort"=w249:refnum<visa-resource-name>)
            n87 = disable-structure shown="Enabled" {
              disable-tunnel: w249 -> [w260 _]
              disable-tunnel: [w257 TRUE] -> w248
              frame #0 {
                n88 = property class="Instr"(reference=w260) -> ("Baud"=w259:u32)  [unwired: 1 in, 2 out]
                n89 = Not Equal?(x=w259, y=u32 19200) -> (x != y?=w257:bool)
              }
              frame #1 {
              }
            }
            n90 = case shown="True" w248 {
              tunnel: [w268 w271] -> w247
              tunnel: [w269 w270] -> w244
              tunnel: w242 -> [w268 w273]
              tunnel: w249 -> [w269 w272]
              frame #0 {
              }
              frame #1 {
                w279 = u16 0 items=["None", "XON/XOFF", "RTS/CTS", "XON/XOFF & RTS/CTS", "DTR/DSR", "XON/XOFF & DTR/DSR"] ("flow control (0:none)")
                w278 = u16 10 items=["1.0"=10, "1.5"=15, "2.0"=20] ("stop bits (10: 1 bit)")
                n91 = call-poly "VISA Configure Serial Port"("VISA resource name"=w272, "timeout (10sec)"=u32 150, "Enable Termination\nChar (T)"=FALSE ("Enable Termination\nChar (T)"), "baud rate (9600)"=u32 19200, "data bits (8)"=u16 8, "parity (0:none)"=enum16{"None", "Odd", "Even", "Mark", "Space"}."None", "error in (no error)"=w273, "stop bits (10: 1 bit)"=w278, "flow control (0:none)"=w279) -> ("VISA resource name out"=w270:refnum<visa-resource-name>, "error out"=w271:errorcluster)  [unwired: 5 in]
              }
            }
            n92 = disable-structure shown="Enabled" {
              disable-tunnel: w244 -> [w254 w256]
              disable-tunnel: [w253 w256] -> w243
              disable-tunnel: [w252 u32 1 ("Bytes at Port")] -> w241
              frame #0 {
                n93 = property class="Instr"(reference=w254) -> (reference out=w253:refnum<visa-resource-name>, "Serial Settings:Number of Bytes at Serial Port"=w252:u32)  [unwired: 1 in, 1 out]
              }
              frame #1 {
              }
            }
            n94 = case shown="1, Default" w241 {
              tunnel: w247 -> [w263 w267]
              tunnel: [w263 w266] -> w246
              tunnel: [w262 w265] -> w245
              tunnel: w243 -> [w262 w264]
              frame #0 {
              }
              frame #1 {
                n95 = VISA Clear(VISA resource name=w264, error in (no error)=w267) -> (VISA resource name out=w265:refnum<visa-resource-name>, error out=w266:errorcluster)
              }
            }
            n96 = Bundle By Name(cluster=w251, "ComPort"=w245) -> (w250:T4)
          }
        }
        n97 = call <vilib>:"Add State(s) to Queue__jki_lib_state_machine.vi"("State(s) in (\"\")"=w229) -> ("States Out"=w228:string)  [unwired: 14 in]
      }
      frame #18 {
        w285 = u8 227  # ETX
        w288 = u8 226  # STX
        n98 = Unbundle By Name(w302) -> ("ComPort"=w301:refnum<visa-resource-name>)
        n99 = call "HEWH_DSM_CMD.vi"("Command"="Command") -> ("CMD Array"=w290:u8[])  [unwired: 10 in]
        n100 = Array Size(array=w290) -> (size(s)=w296:i32)
        n101 = Array Size(array="Command Data") -> (size(s)=w294:i32)
        n102 = Compound Arithmetic op=ADD(7 ("x"), w296, w294) -> (w292:i32)
        n103 = To Unsigned Byte Integer(number=w292) -> (unsigned 8bit integer=w293:u8)
        n104 = Build Array (concatenate)("Destination Address", w293, "Source Address", w290, "Command Data") -> (w287:u8[])
        n105 = call "crc16-ccitt (x1021).vi"("unsigned byte array"=w287) -> ("CRC"=w286:u8[])  [unwired: 9 in, 1 out]
        n106 = flat-sequence {
          tunnel: [w333] -> w282
          frame #0 {
            n107 = Tick Count (ms)() -> (millisecond timer value=w333:u32)
          }
        }
        n108 = Build Array (concatenate)(w288, w287, w286, w285) -> (w284:u8[])
        "Command" <- w284
        n109 = To Long Integer(number=w282) -> (32bit integer=→"tStart":i32)
        n110 = disable-structure shown="Enabled" {
          disable-tunnel: w301 -> [w311 w332]
          disable-tunnel: w300 -> [w309 w331]
          disable-tunnel: [w308 w328] -> w299
          disable-tunnel: w284 -> [w307 w326]
          disable-tunnel: [w306 w323] -> w283
          disable-tunnel: w282 -> [w305 _]
          frame #0 {
            n111 = for {
              tunnel: w311 -> [w322]
              tunnel: w307 -> [w318] mode=indexing
              tunnel: [w315] -> w310 mode=indexing
              shift-right: [w314] -> w308
              shift-left: w309 -> [w313]
              tunnel: w305 -> [_]
              n112 = Build Array(w318) -> (w319:u8[])
              n113 = Byte Array To String(unsigned byte array=w319) -> (string=w316:string)
              n114 = VISA Write(VISA resource name=w322, write buffer=w316, error in (no error)=w313) -> (VISA resource name out=w321:refnum<visa-resource-name>, error out=w312:errorcluster)  [unwired: 1 out]
              n115 = VISA Read(VISA resource name=w321, byte count=u32 1, error in (no error)=w312) -> (read buffer=w317:string, error out=w314:errorcluster)  [unwired: 2 out]
              n116 = Equal?(x=w316, y=w317) -> (x = y?=w315:bool)
            }
            n117 = And Array Elements(Boolean array=w310) -> (logical AND=w306:bool)
          }
          frame #1 {
            n118 = Byte Array To String(unsigned byte array=w326) -> (string=w324:string)
            n119 = VISA Write(VISA resource name=w332, write buffer=w324, error in (no error)=w331) -> (VISA resource name out=w329:refnum<visa-resource-name>, error out=w330:errorcluster)  [unwired: 1 out]
            n120 = Array Size(array=w326) -> (size(s)=w327:i32)
            n121 = VISA Read(VISA resource name=w329, byte count=w327, error in (no error)=w330) -> (read buffer=w325:string, error out=w328:errorcluster)  [unwired: 2 out]
            n122 = Equal?(x=w324, y=w325) -> (x = y?=w323:bool)
          }
        }
        "WriteOK" <- w283
        n123 = call <vilib>:"Add State(s) to Queue__jki_lib_state_machine.vi"("State(s) in (\"\")"=w304) -> ("States Out"=w303:string)  [unwired: 14 in]
      }
      frame #19 {
        # "Your code here.\n(You can make a copy of, or modify, this frame)"
        n124 = Unbundle By Name(w340) -> ("ComPort"=w339:refnum<visa-resource-name>)
        n125 = for {
          tunnel: w339 -> [w353]
          tunnel: "Random Data" -> [w349] mode=indexing
          tunnel: [w346] -> w338 mode=indexing
          shift-right: [w345] -> w336
          shift-left: w337 -> [w344]
          n126 = Build Array(w349) -> (w350:u8[])
          n127 = Byte Array To String(unsigned byte array=w350) -> (string=w347:string)
          n128 = VISA Write(VISA resource name=w353, write buffer=w347, error in (no error)=w344) -> (VISA resource name out=w352:refnum<visa-resource-name>, error out=w343:errorcluster)  [unwired: 1 out]
          n129 = VISA Read(VISA resource name=w352, byte count=u32 1, error in (no error)=w343) -> (read buffer=w348:string, error out=w345:errorcluster)  [unwired: 2 out]
          n130 = Equal?(x=w347, y=w348) -> (x = y?=w346:bool)
        }
        n131 = And Array Elements(Boolean array=w338) -> (logical AND=w334:bool)
        n132 = local write "WriteOK"(w334) -> ()
        n133 = call <vilib>:"Add State(s) to Queue__jki_lib_state_machine.vi"("State(s) in (\"\")"=w342) -> ("States Out"=w341:string)  [unwired: 14 in]
      }
      frame #20 {
        # "Template Separator\n(You can make a copy of, or modify, this frame)"
        n134 = call <vilib>:"Add State(s) to Queue__jki_lib_state_machine.vi"("State(s) in (\"\")"=w357) -> ("States Out"=w356:string)  [unwired: 14 in]
      }
      frame #21 {
        w358 = u8[] [] ("ReadArray")
        # "Your code here.\n(You can make a copy of, or modify, this frame)"
        n135 = Bundle By Name(cluster=w361, "ReadArray"=w358, "CRCArray"=w358) -> (w360:T4)
        n136 = local write "ReadArray"(w358) -> ()
        n137 = call <vilib>:"Add State(s) to Queue__jki_lib_state_machine.vi"("State(s) in Front (\"\")"="ReadData: ACK" ("State(s) in Front (\"\")"), "State(s) in (\"\")"=w364) -> ("States Out"=w363:string)  [unwired: 13 in]
      }
      frame #22 {
        w366 = u8 225  # ACK
        # "Read ACK Byte"
        n138 = Unbundle By Name(w378) -> ("ComPort"=w380:refnum<visa-resource-name>, "ReadArray"=w365:u8[])
        n139 = local write "ReadArray"(w365) -> ()
        n140 = VISA Read(VISA resource name=w380, byte count=u32 1, error in (no error)=w371) -> (read buffer=w375:string, error out=w369:errorcluster)  [unwired: 2 out]
        n141 = String To Byte Array(string=w375) -> (unsigned byte array=w374:u8[])
        n142 = Index Array(array=w374, index=0) -> (element=w372:u8)
        n143 = Build Array (concatenate)(w365, w374) -> (w379:u8[])
        n144 = Equal?(x=w372, y=w366) -> (x = y?=w370:bool)
        "WriteACK" <- w370
        n145 = Bundle By Name(cluster=w378, "ReadArray"=w379) -> (w377:T4)
        n146 = case shown="True" w370 {
          tunnel: w369 -> [w384 w388]
          tunnel: [w386 w388] -> w368
          tunnel: ["" ("State(s) in Front (\"\")") "ReadData: STX" ("State(s) in Front (\"\")")] -> w367
          frame #0 {
            n147 = call "Error Bool Enumerator.vi"("Error Enum"=HEWH_Error_Enumeration."GEA2 Send ACK Mismatch", "Error In"=w384) -> ("Error Out"=w386:errorcluster)  [unwired: 7 in]
          }
          frame #1 {
          }
        }
        n148 = call <vilib>:"Add State(s) to Queue__jki_lib_state_machine.vi"("State(s) in Front (\"\")"=w367, "State(s) in (\"\")"=w382) -> ("States Out"=w381:string)  [unwired: 13 in]
      }
      frame #23 {
        w398 = u8 224  # ESC
        # "Read Destination byte.  If its your message, than continue to length, otherwise, read the rest of the message."
        n149 = Unbundle By Name(w411) -> ("ComPort"=w391:refnum<visa-resource-name>, "ReadArray"=w389:u8[])
        n150 = VISA Read(VISA resource name=w391, byte count=u32 1, error in (no error)=w405) -> (read buffer=w408:string, error out=w393:errorcluster)  [unwired: 2 out]
        n151 = String To Byte Array(string=w408) -> (unsigned byte array=w395:u8[])
        n152 = Index Array(array=w395, index=0) -> (element=w400:u8)
        n153 = local write "ReadArray"(w389) -> ()
        n154 = Equal?(x=w400, y=w398) -> (x = y?=w397:bool)
        n155 = case shown="True" w397 {
          tunnel: [w416 w417] -> w396
          tunnel: w395 -> [w416 w424]
          tunnel: [w415 w418] -> w394
          tunnel: w389 -> [w415 w425]
          tunnel: w393 -> [w414 w421]
          tunnel: [w414 w420] -> w392
          tunnel: w391 -> [_ w419]
          frame #0 {
          }
          frame #1 {
            n156 = VISA Read(VISA resource name=w419, byte count=u32 1, error in (no error)=w421) -> (read buffer=w423:string, error out=w420:errorcluster)  [unwired: 2 out]
            n157 = String To Byte Array(string=w423) -> (unsigned byte array=w417:u8[])
            n158 = Build Array (concatenate)(w425, w424) -> (w418:u8[])
          }
        }
        n159 = Build Array (concatenate)(w394, w396) -> (w390:u8[])
        n160 = local read "Source Address"() -> (w401:u8)
        n161 = Index Array(array=w396, index=0) -> (element=w406:u8)
        n162 = Bundle By Name(cluster=w411, "ReadArray"=w390, "CRCArray"=w396) -> (w410:T4)
        n163 = Equal?(x=w406, y=w401) -> (x = y?=w404:bool)
        n164 = case shown="False" w404 {
          tunnel: w392 -> [w429 w431]
          tunnel: [w427 w431] -> w403
          tunnel: ["ReadData: Rest" ("State(s) in Front (\"\")") "ReadData: Length" ("State(s) in Front (\"\")")] -> w402
          frame #0 {
            n165 = call <vilib>:"Merge Errors.vi"("error in 2 (no error)"=errorcluster {"status"=FALSE, "code"=7000, "source"="Message not for Me"}, "error in 1 (no error)"=w429) -> ("error out"=w427:errorcluster)  [unwired: 5 in]
          }
          frame #1 {
          }
        }
        n166 = call <vilib>:"Add State(s) to Queue__jki_lib_state_machine.vi"("State(s) in Front (\"\")"=w402, "State(s) in (\"\")"=w413) -> ("States Out"=w412:string)  [unwired: 13 in]
      }
      frame #24 {
        w446 = u8 224  # ESC
        # "Your code here.\n(You can make a copy of, or modify, this frame)"
        n167 = Unbundle By Name(w457) -> ("ComPort"=w440:refnum<visa-resource-name>, "ReadArray"=w438:u8[], "CRCArray"=w432:u8[])
        n168 = VISA Read(VISA resource name=w440, byte count=u32 1, error in (no error)=w452) -> (read buffer=w454:string, error out=w442:errorcluster)  [unwired: 2 out]
        n169 = String To Byte Array(string=w454) -> (unsigned byte array=w444:u8[])
        n170 = local write "ReadArray"(w438) -> ()
        n171 = Index Array(array=w444, index=0) -> (element=w448:u8)
        n172 = Equal?(x=w448, y=w446) -> (x = y?=w445:bool)
        n173 = case shown="True" w445 {
          tunnel: [w463 w464] -> w433
          tunnel: w444 -> [w463 w471]
          tunnel: [w462 w465] -> w443
          tunnel: w438 -> [w462 w472]
          tunnel: w442 -> [w461 w468]
          tunnel: [w461 w467] -> w441
          tunnel: w440 -> [_ w466]
          frame #0 {
          }
          frame #1 {
            n174 = VISA Read(VISA resource name=w466, byte count=u32 1, error in (no error)=w468) -> (read buffer=w470:string, error out=w467:errorcluster)  [unwired: 2 out]
            n175 = String To Byte Array(string=w470) -> (unsigned byte array=w464:u8[])
            n176 = Build Array (concatenate)(w472, w471) -> (w465:u8[])
          }
        }
        n177 = Index Array(array=w433, index=0) -> (element=w437:u8)
        n178 = Build Array (concatenate)(w443, w433) -> (w458:u8[])
        n179 = Subtract(x=w437, y=u8 6) -> (x-y=w435:u8)
        n180 = Build Array (concatenate)(w432, w433) -> (w434:u8[])
        n181 = Less Or Equal?(x=w435, y=u8 0 ("0")) -> (x <= y?=w451:bool)
        n182 = Bundle By Name(cluster=w457, "ReadArray"=w458, "CRCArray"=w434, "Bytes Remaining"=w435) -> (w456:T4)
        n183 = case shown="True" w451 {
          tunnel: w441 -> [w474 w478]
          tunnel: [w474 w476] -> w450
          tunnel: ["ReadData: Bytes" ("State(s) in Front (\"\")") "ReadData: Rest" ("State(s) in Front (\"\")")] -> w449
          frame #0 {
          }
          frame #1 {
            n184 = call <vilib>:"Merge Errors.vi"("error in 2 (no error)"=errorcluster {"status"=FALSE, "code"=7000, "source"="0 Length"}, "error in 1 (no error)"=w478) -> ("error out"=w476:errorcluster)  [unwired: 5 in]
          }
        }
        n185 = call <vilib>:"Add State(s) to Queue__jki_lib_state_machine.vi"("State(s) in Front (\"\")"=w449, "State(s) in (\"\")"=w460) -> ("States Out"=w459:string)  [unwired: 13 in]
      }
      frame #25 {
        w492 = u8 224  # ESC
        # "Your code here.\n(You can make a copy of, or modify, this frame)"
        n186 = Unbundle By Name(w501) -> ("ComPort"=w486:refnum<visa-resource-name>, "ReadArray"=w482:u8[], "Bytes Remaining"=w484:u8, "CRCArray"=w479:u8[])
        n187 = VISA Read(VISA resource name=w486, byte count=u32 1, error in (no error)=w497) -> (read buffer=w498:string, error out=w488:errorcluster)  [unwired: 2 out]
        n188 = String To Byte Array(string=w498) -> (unsigned byte array=w490:u8[])
        n189 = Index Array(array=w490, index=0) -> (element=w494:u8)
        n190 = Equal?(x=w494, y=w492) -> (x = y?=w491:bool)
        n191 = case shown="True" w491 {
          tunnel: [w507 w508] -> w481
          tunnel: w490 -> [w507 w515]
          tunnel: [w506 w509] -> w489
          tunnel: w482 -> [w506 w516]
          tunnel: w488 -> [w505 w512]
          tunnel: [w505 w511] -> w487
          tunnel: w486 -> [_ w510]
          frame #0 {
          }
          frame #1 {
            n192 = VISA Read(VISA resource name=w510, byte count=u32 1, error in (no error)=w512) -> (read buffer=w514:string, error out=w511:errorcluster)  [unwired: 2 out]
            n193 = String To Byte Array(string=w514) -> (unsigned byte array=w508:u8[])
            n194 = Build Array (concatenate)(w516, w515) -> (w509:u8[])
          }
        }
        n195 = local write "ReadArray"(w482) -> ()
        n196 = Decrement(x=w484) -> (x-1=w483:u8)
        n197 = Build Array (concatenate)(w479, w481) -> (w480:u8[])
        n198 = Build Array (concatenate)(w489, w481) -> (w502:u8[])
        n199 = Greater Than 0?(x=w483) -> (x > 0?=w485:bool)
        n200 = Bundle By Name(cluster=w501, "ReadArray"=w502, "CRCArray"=w480, "Bytes Remaining"=w483) -> (w500:T4)
        n201 = case shown="False" w485 {
          tunnel: w487 -> [w520 w522]
          tunnel: [w518 w522] -> w496
          tunnel: ["ReadData: CRC1" ("State(s) in Front (\"\")") "ReadData: Bytes" ("State(s) in Front (\"\")")] -> w495
          frame #0 {
            n202 = call <vilib>:"Merge Errors.vi"("error in 2 (no error)"=errorcluster {"status"=FALSE, "code"=7000, "source"="0 Length"}, "error in 1 (no error)"=w520) -> ("error out"=w518:errorcluster)  [unwired: 5 in]
          }
          frame #1 {
          }
        }
        n203 = call <vilib>:"Add State(s) to Queue__jki_lib_state_machine.vi"("State(s) in Front (\"\")"=w495, "State(s) in (\"\")"=w504) -> ("States Out"=w503:string)  [unwired: 13 in]
      }
      frame #26 {
        w531 = u8 224  # ESC
        # "Your code here.\n(You can make a copy of, or modify, this frame)"
        n204 = Unbundle By Name(w539) -> ("ComPort"=w525:refnum<visa-resource-name>, "ReadArray"=w527:u8[])
        n205 = VISA Read(VISA resource name=w525, byte count=u32 1, error in (no error)=w535) -> (read buffer=w536:string, error out=w526:errorcluster)  [unwired: 2 out]
        n206 = String To Byte Array(string=w536) -> (unsigned byte array=w529:u8[])
        n207 = Index Array(array=w529, index=0) -> (element=w533:u8)
        n208 = Equal?(x=w533, y=w531) -> (x = y?=w530:bool)
        n209 = case shown="True" w530 {
          tunnel: [w545 w546] -> w524
          tunnel: w529 -> [w545 w553]
          tunnel: [w544 w547] -> w528
          tunnel: w527 -> [w544 w554]
          tunnel: w526 -> [w543 w550]
          tunnel: [w543 w549] -> w523
          tunnel: w525 -> [_ w548]
          frame #0 {
          }
          frame #1 {
            n210 = VISA Read(VISA resource name=w548, byte count=u32 1, error in (no error)=w550) -> (read buffer=w552:string, error out=w549:errorcluster)  [unwired: 2 out]
            n211 = String To Byte Array(string=w552) -> (unsigned byte array=w546:u8[])
            n212 = Build Array (concatenate)(w554, w553) -> (w547:u8[])
          }
        }
        n213 = Build Array (concatenate)(w528, w524) -> (w540:u8[])
        n214 = Bundle By Name(cluster=w539, "ReadArray"=w540, "CRCRead"=w524) -> (w538:T4)
        n215 = call <vilib>:"Add State(s) to Queue__jki_lib_state_machine.vi"("State(s) in Front (\"\")"="ReadData: CRC2" ("State(s) in Front (\"\")"), "State(s) in (\"\")"=w542) -> ("States Out"=w541:string)  [unwired: 13 in]
      }
      frame #27 {
        w566 = u8 224  # ESC
        # "Your code here.\n(You can make a copy of, or modify, this frame)"
        n216 = Unbundle By Name(w574) -> ("ComPort"=w561:refnum<visa-resource-name>, "ReadArray"=w557:u8[], "CRCRead"=w556:u8[])
        n217 = VISA Read(VISA resource name=w561, byte count=u32 1, error in (no error)=w570) -> (read buffer=w571:string, error out=w562:errorcluster)  [unwired: 2 out]
        n218 = String To Byte Array(string=w571) -> (unsigned byte array=w564:u8[])
        n219 = Index Array(array=w564, index=0) -> (element=w568:u8)
        n220 = Equal?(x=w568, y=w566) -> (x = y?=w565:bool)
        n221 = case shown="True" w565 {
          tunnel: [w579 w580] -> w558
          tunnel: w564 -> [w579 w587]
          tunnel: [w578 w581] -> w563
          tunnel: w557 -> [w578 w588]
          tunnel: w562 -> [w577 w584]
          tunnel: [w577 w583] -> w560
          tunnel: w561 -> [_ w582]
          frame #0 {
          }
          frame #1 {
            n222 = VISA Read(VISA resource name=w582, byte count=u32 1, error in (no error)=w584) -> (read buffer=w586:string, error out=w583:errorcluster)  [unwired: 2 out]
            n223 = String To Byte Array(string=w586) -> (unsigned byte array=w580:u8[])
            n224 = Build Array (concatenate)(w588, w587) -> (w581:u8[])
          }
        }
        n225 = local write "ReadArray"(w557) -> ()
        n226 = Build Array (concatenate)(w563, w558) -> (w559:u8[])
        n227 = Build Array (concatenate)(w556, w558) -> (w555:u8[])
        n228 = Bundle By Name(cluster=w574, "ReadArray"=w559, "CRCRead"=w555) -> (w573:T4)
        n229 = local write "CRCRead"(w555) -> ()
        n230 = call <vilib>:"Add State(s) to Queue__jki_lib_state_machine.vi"("State(s) in Front (\"\")"="ReadData: CheckCRC" ("State(s) in Front (\"\")"), "State(s) in (\"\")"=w576) -> ("States Out"=w575:string)  [unwired: 13 in]
      }
      frame #28 {
        # "Your code here.\n(You can make a copy of, or modify, this frame)"
        n231 = Unbundle By Name(w591) -> ("CRCRead"=w596:u8[], "CRCArray"=w593:u8[])
        "DataReturned" <- w593
        n232 = call "crc16-ccitt (x1021).vi"("error in (no error)"=w597, "unsigned byte array"=w593) -> ("error out (dup)"=w594:errorcluster, "CRC"=w592:u8[])  [unwired: 8 in]
        n233 = Equal?(x=w596, y=w592) -> (x = y?=w589:bool)
        "CRC Match" <- w589
        n234 = case shown="False" w589 {
          tunnel: ["ReadData: Rest" ("State(s) in Front (\"\")") "ReadData: ETX" ("State(s) in Front (\"\")")] -> w598
          tunnel: [w604 w606] -> w595
          tunnel: w594 -> [w603 w606]
          frame #0 {
            n235 = call "Error Bool Enumerator.vi"("Error Enum"=HEWH_Error_Enumeration."GEA2 CRC Mismatch", "Error In"=w603, "Error?"=TRUE) -> ("Error Out"=w604:errorcluster)  [unwired: 6 in]
          }
          frame #1 {
          }
        }
        n236 = Bundle By Name(cluster=w591, "CRC"=w589) -> (w590:T4)
        n237 = call <vilib>:"Add State(s) to Queue__jki_lib_state_machine.vi"("State(s) in Front (\"\")"=w598, "State(s) in (\"\")"=w600) -> ("States Out"=w599:string)  [unwired: 13 in]
      }
      frame #29 {
        w608 = u8 226  # STX
        # "Your code here.\n(You can make a copy of, or modify, this frame)"
        n238 = Unbundle By Name(w620) -> ("ComPort"=w623:refnum<visa-resource-name>, "ReadArray"=w622:u8[])
        n239 = VISA Read(VISA resource name=w623, byte count=u32 1, error in (no error)=w618) -> (read buffer=w612:string, error out=w616:errorcluster)  [unwired: 2 out]
        n240 = String To Byte Array(string=w612) -> (unsigned byte array=w611:u8[])
        n241 = Index Array(array=w611, index=0) -> (element=w609:u8)
        n242 = Build Array (concatenate)(w622, w611) -> (w621:u8[])
        n243 = Equal?(x=w609, y=w608) -> (x = y?=w617:bool)
        n244 = Bundle By Name(cluster=w620, "ReadArray"=w621) -> (w619:T4)
        n245 = case shown="True" w617 {
          tunnel: w616 -> [w628 w632]
          tunnel: [w627 w632] -> w615
          tunnel: ["ReadData: Rest" ("State(s) in Front (\"\")") "ReadData: Destination" ("State(s) in Front (\"\")")] -> w614
          frame #0 {
            n246 = call "Error Bool Enumerator.vi"("Error Enum"=HEWH_Error_Enumeration."GEA2 STX", "Error In"=w628, "Error?"=TRUE) -> ("Error Out"=w627:errorcluster)  [unwired: 6 in]
          }
          frame #1 {
          }
        }
        n247 = call <vilib>:"Add State(s) to Queue__jki_lib_state_machine.vi"("State(s) in Front (\"\")"=w614, "State(s) in (\"\")"=w625) -> ("States Out"=w624:string)  [unwired: 13 in]
      }
      frame #30 {
        w633 = u8 227  # ETX
        # "Your code here.\n(You can make a copy of, or modify, this frame)"
        n248 = Unbundle By Name(w645) -> ("ComPort"=w648:refnum<visa-resource-name>, "ReadArray"=w647:u8[])
        n249 = VISA Read(VISA resource name=w648, byte count=u32 1, error in (no error)=w643) -> (read buffer=w637:string, error out=w641:errorcluster)  [unwired: 2 out]
        n250 = String To Byte Array(string=w637) -> (unsigned byte array=w636:u8[])
        n251 = Index Array(array=w636, index=0) -> (element=w634:u8)
        n252 = Build Array (concatenate)(w647, w636) -> (w646:u8[])
        n253 = Equal?(x=w634, y=w633) -> (x = y?=w642:bool)
        n254 = Bundle By Name(cluster=w645, "ReadArray"=w646) -> (w644:T4)
        n255 = case shown="True" w642 {
          tunnel: w641 -> [w653 w657]
          tunnel: [w655 w657] -> w640
          tunnel: ["ReadData: Rest" ("State(s) in Front (\"\")") "ReadData: SendACK" ("State(s) in Front (\"\")")] -> w639
          frame #0 {
            n256 = call "Error Bool Enumerator.vi"("Error Enum"=HEWH_Error_Enumeration."GEA2 ETX", "Error In"=w653, "Error?"=TRUE) -> ("Error Out"=w655:errorcluster)  [unwired: 6 in]
          }
          frame #1 {
          }
        }
        n257 = call <vilib>:"Add State(s) to Queue__jki_lib_state_machine.vi"("State(s) in Front (\"\")"=w639, "State(s) in (\"\")"=w650) -> ("States Out"=w649:string)  [unwired: 13 in]
      }
      frame #31 {
        n258 = Unbundle By Name(w665) -> ("ComPort"=w662:refnum<visa-resource-name>, "ReadArray"=w666:u8[])
        n259 = disable-structure shown="Enabled" {
          disable-tunnel: w662 -> [w672 w674]
          disable-tunnel: [w671 w674] -> w661
          disable-tunnel: [w670 u32 100 ("Bytes at Port")] -> w658
          frame #0 {
            n260 = property class="Instr"(reference=w672) -> (reference out=w671:refnum<visa-resource-name>, "Serial Settings:Number of Bytes at Serial Port"=w670:u32)  [unwired: 1 in, 1 out]
          }
          frame #1 {
          }
        }
        n261 = VISA Read(VISA resource name=w661, byte count=w658) -> (read buffer=w660:string)  [unwired: 1 in, 3 out]
        n262 = String To Byte Array(string=w660) -> (unsigned byte array=w659:u8[])
        n263 = Build Array (concatenate)(w666, w659) -> (w663:u8[])
        n264 = local write "ReadArray"(w663) -> ()
        n265 = Bundle By Name(cluster=w665, "ReadArray"=w663) -> (w664:T4)
        n266 = call <vilib>:"Add State(s) to Queue__jki_lib_state_machine.vi"("State(s) in (\"\")"=w669) -> ("States Out"=w668:string)  [unwired: 14 in]
      }
      frame #32 {
        w685 = u8 225  # ACK
        n267 = Unbundle By Name(w692) -> ("ComPort"=w676:refnum<visa-resource-name>)
        n268 = property class="Instr"(reference=w676) -> ("Serial Settings:Number of Bytes at Serial Port"=→"Serial Settings:Number of Bytes at Serial Port":u32)  [unwired: 1 in, 2 out]
        n269 = Build Array(w685) -> (w688:u8[])
        n270 = Byte Array To String(unsigned byte array=w688) -> (string=w687:string)
        n271 = VISA Write(VISA resource name=w676, write buffer=w687, error in (no error)=w691) -> (VISA resource name out=w690:refnum<visa-resource-name>, error out=w686:errorcluster)  [unwired: 1 out]
        n272 = VISA Read(VISA resource name=w690, byte count=u32 1, error in (no error)=w686) -> (read buffer=w683:string, error out=w684:errorcluster)  [unwired: 2 out]
        n273 = Equal?(x=w687, y=w683) -> (x = y?=w680:bool)
        "Read_ACK" <- w680
        n274 = String To Byte Array(string=w683) -> (unsigned byte array=→"ACK(E1?)":u8[])
        n275 = Not(x=w680) -> (.not. x?=w679:bool)
        n276 = call "Error Bool Enumerator.vi"("Error Enum"=HEWH_Error_Enumeration."GEA2 Send ACK Mismatch", "Error In"=w684, "Error?"=w679) -> ("Error Out"=w678:errorcluster)  [unwired: 6 in]
        n277 = case shown="No Error" w678 {
          tunnel: ["Macro: Exit" ("State(s) in Front (\"\")") "ReadData: Rest" ("State(s) in Front (\"\")")] -> w677
          frame #0 {
          }
          frame #1 {
          }
        }
        n278 = call <vilib>:"Add State(s) to Queue__jki_lib_state_machine.vi"("State(s) in Front (\"\")"=w677, "State(s) in (\"\")"=w694) -> ("States Out"=w693:string)  [unwired: 13 in]
      }
    }
    n279 = local write "Error Out"(w30) -> ()
    n280 = flat-sequence {
      tunnel: [w42] -> w29
      tunnel: w30 -> [_]
      frame #0 {
        n281 = Tick Count (ms)() -> (millisecond timer value=w42:u32)
      }
    }
  }
  "State Array" <- w17
  n282 = flat-sequence {
    tunnel: [w700] -> w13
    tunnel: w12 -> [w699]
    frame #0 {
      n283 = local read "tStart"() -> (w698:i32)
      n284 = To Long Integer(number=w699) -> (32bit integer=w697:i32[])
      n285 = Subtract(x=w697, y=w698) -> (x-y=w700:i32[])
    }
  }
  n286 = flat-sequence {
    tunnel: [w704] -> w3
    tunnel: w18 -> [w703]
    tunnel: w2 -> [w702]
    frame #0 {
      n287 = Unbundle By Name(w702) -> ("Error Out Flag"=w701:bool)
      n288 = case shown="True" w701 {
        tunnel: w703 -> [w705 w708]
        tunnel: [w705 w706] -> w704
        frame #0 {
        }
        frame #1 {
          n289 = Bundle By Name(cluster=w708, "status"=TRUE) -> (w706:errorcluster)
        }
      }
    }
  }
  n290 = To Long Integer(number=w9) -> (32bit integer=w8:i32)
  n291 = Delete From Array(array=w13, length=1, index=0) -> (deleted portion=w5:i32[], array with subset deleted=w14:i32[])
  n292 = Build Array(w8) -> (w6:i32[])
  n293 = for {
    tunnel: w14 -> [w711] mode=indexing
    tunnel: w13 -> [w710] mode=indexing
    tunnel: [w709] -> w11 mode=indexing
    n294 = Subtract(x=w711, y=w710) -> (x-y=w709:i32)
  }
  n295 = Subtract(x=w5, y=w6) -> (x-y=w7:i32[])
  n296 = Build Array (concatenate)(w7, w11) -> (→"Diff Time":i32[])
  n297 = Unbundle By Name(w2) -> ("CRC"=w1:bool)
  n298 = disable-structure shown="Enabled" {
    disable-tunnel: [w714 w724] -> w4
    disable-tunnel: w3 -> [w713 w724]
    disable-tunnel: w1 -> [w712 _]
    frame #0 {
      w719 = 7000  # UserOffset
      # "Patch for double read of ICP"
      n299 = To Long Integer(number=HEWH_Error_Enumeration."GEA2 Send ACK Mismatch" ("Error Enum")) -> (32bit integer=w717:i32)
      n300 = Unbundle By Name(w713) -> ("code"=w721:i32)  [unwired: 1 out]
      n301 = Add(x=w717, y=w719) -> (x+y=w718:i32)
      n302 = Equal?(x=w721, y=w718) -> (x = y?=w716:bool)
      n303 = And(x=w712, y=w716) -> (x .and. y?=w715:bool)
      n304 = case shown="False" w715 {
        tunnel: [w722 errorcluster {"status"=FALSE, "code"=0, "source"="ACK"} ("Error Out")] -> w714
        tunnel: w713 -> [w722 _]
        frame #0 {
        }
        frame #1 {
        }
      }
    }
    frame #1 {
    }
  }
  "Error Out" <- w4
  "Time Array" <- w13
